vi "SynchroResolver Simulation RtDmap.vi"() -> ()   [LabVIEW 8.6]
uses:
  vi.lib/UeiDaq/UeiDaqReadOneScaledScan.vi
  vi.lib/UeiDaq/UeiDaqWriteOneScaledScan.vi
  vi.lib/UeiDaq/UeiDaqCreateSynchroResolverSession.vi
  vi.lib/UeiDaq/UeiDaqCreateSimulatedSynchroResolverSession.vi
  vi.lib/UeiDaq/UeiDaqConfigureTimingForRTDMapIO.vi
panel:
  in  "Mode":enum16{"Synchro", "Resolver"}(ring)
  out "Measured Excitation Frequency":dbl[](array[numeric])
  out "Measured Excitation Amplitude":dbl[](array[numeric])
  in  "Excitation frequency":dbl
  in  "Excitation amplitude":dbl
  in  "Simulated Synchro/Resolver position in Radians":dbl(slide)
  in  "Simulated Output Resource":string
  out "Measured LVDT position":dbl[][](graph)
  in  "RTDmap Refresh \nRate (Hz)":u32
  in  "stop":bool
  in  "Input Resource":string
  # "Synchro/Resolver Simulation"
  # "This example takes advantage of the Synchro/Resolver simulation capability on the AI-255.It Simulates a Synchro or a Resolver out of channel 1 and measures it back on channel 0. You need to connect the folowing pins:\nCh0 IN A- <--> Ch1 OUT A-\nCh0 IN A+ <--> Ch1 OUT A+\nCh0 IN B- <--> Ch1 OUT B-\nCh0 IN B+ <--> Ch1 OUT B+\nCh0 IN C- <--> Ch1 OUT C-\nCh0 IN C+ <--> Ch1 OUT C+\nCh0 OUT D- <--> Ch1 IN D-\nCh0 OUT D+ <--> Ch1 IN D+"
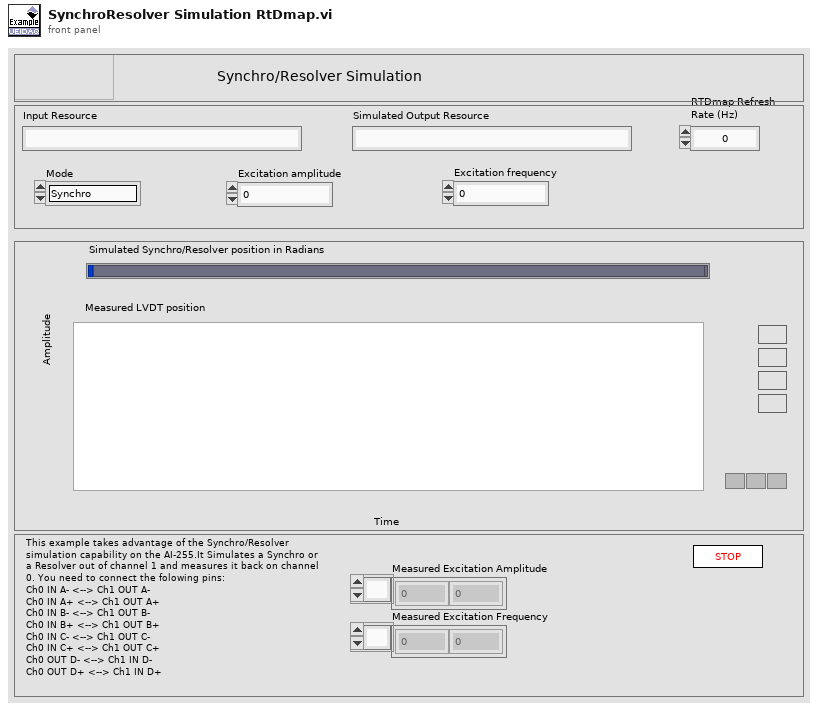
[diagram p1: front panel]
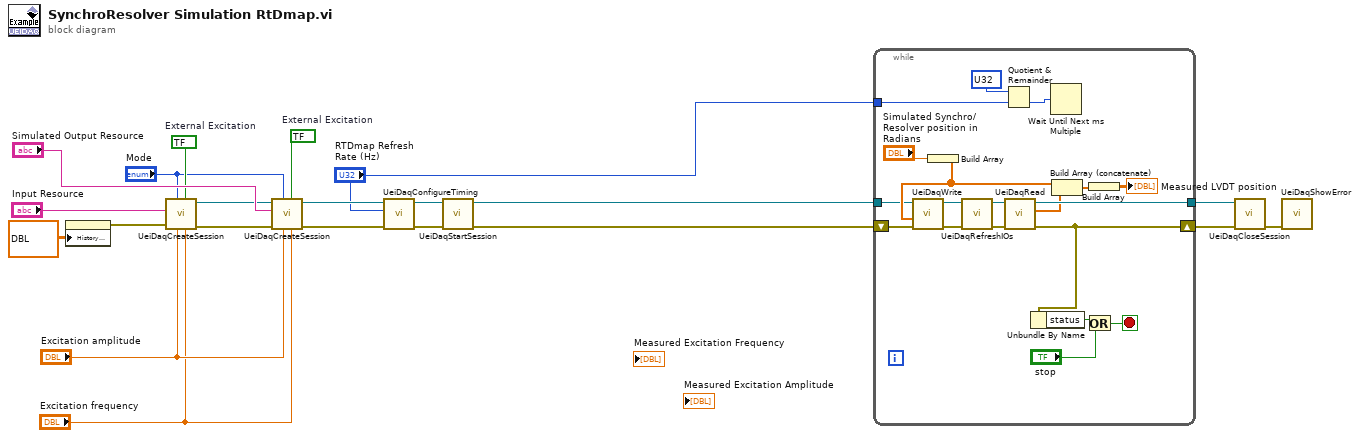
[diagram p0: block diagram]
diagram:
  w10 = bool ?  # External Excitation
  w12 = bool ?  # External Excitation
  n1 = property on="Measured LVDT position" class="WFChart (strict)"("History Data"=dbl[][] ?) -> (error out=w16:errorcluster)  [unwired: 2 in, 1 out]
  n2 = call-poly "UeiDaqCreateSession.vi"("Excitation frequency"="Excitation frequency", "External Excitation"=w12, "Excitation voltage"="Excitation amplitude", "Mode"="Mode", "error in (no error)"=w16, "Resource"="Input Resource") -> ("error out"=w7:errorcluster, "UeiDaq Refnum Out"=w8:refnum<k20>)  [unwired: 1 in, 3 out]
  n3 = call-poly "UeiDaqCreateSession.vi"("Excitation frequency"="Excitation frequency", "External Excitation"=w10, "Excitation voltage"="Excitation amplitude", "Mode"="Mode", "error in (no error)"=w7, "Resource"="Simulated Output Resource", "UeiDaq Refnum In"=w8) -> ("error out"=w4:errorcluster, "UeiDaq Refnum Out"=w6:refnum<k20>)  [unwired: 3 out]
  n4 = call-poly "UeiDaqConfigureTiming.vi"("error in (no error)"=w4, "Rate"="RTDmap Refresh \nRate (Hz)", "UeiDaq Refnum In"=w6) -> ("error out"=w15:errorcluster, "UeiDaq Refnum Out"=w5:refnum<k20>)  [unwired: 7 out]
  n5 = call "UeiDaqStartSession.vi"("error in (no error)"=w15, "UeiDaq Refnum In"=w5) -> ("error out"=w1:errorcluster, "UeiDaq Refnum Out"=w2:refnum<k20>)  [unwired: 8 out]
  n6 = while {
    tunnel: [w38] -> w19
    tunnel: w2 -> [w26]
    shift-right: [w32] -> w9
    shift-left: w1 -> [w27]
    tunnel: "RTDmap Refresh \nRate (Hz)" -> [w24]
    stop <- w39 stop-if-true
    n7 = Build Array("Simulated Synchro/Resolver position in Radians") -> (w35:dbl[])
    n8 = call-poly "UeiDaqWrite.vi"("error in (no error)"=w27, "Scaled Data"=w35, "UeiDaq Refnum In"=w26) -> ("error out"=w31:errorcluster, "UeiDaq Refnum Out"=w30:refnum<k20>)  [unwired: 1 in, 6 out]
    n9 = call "UeiDaqRefreshIOs.vi"("error in (no error)"=w31, "UeiDaq Refnum In"=w30) -> ("error out"=w28:errorcluster, "UeiDaq Refnum Out"=w29:refnum<k20>)  [unwired: 8 in]
    n10 = Quotient & Remainder(x=u32 ?, y=w24) -> (floor(x/y)=w23:u32)  [unwired: 1 out]
    n11 = call-poly "UeiDaqRead.vi"("error in (no error)"=w28, "UeiDaq Refnum In"=w29) -> ("error out"=w32:errorcluster, "Scaled Data"=w36:dbl[], "UeiDaq Refnum Out"=w38:refnum<k20>)  [unwired: 7 out]
    n12 = Unbundle By Name(w32) -> ("status"=w37:bool)
    n13 = Wait Until Next ms Multiple(millisecond multiple=w23) -> ()  [unwired: 1 out]
    n14 = Build Array (concatenate)(w35, w36) -> (w34:dbl[])
    n15 = Or(x=w37, y="stop") -> (x .or. y?=w39:bool)
    n16 = Build Array(w34) -> (→"Measured LVDT position":dbl[][])
  }
  n17 = call "UeiDaqCloseSession.vi"("error in (no error)"=w9, "UeiDaq Refnum In"=w19) -> ("error out"=w18:errorcluster)  [unwired: 1 in, 8 out]
  n18 = call "UeiDaqShowError.vi"("error in (no error)"=w18) -> ()  [unwired: 2 in, 9 out]
